vi "应变求平均.vi"(2 "调零采样数":u8=10, 3 "应变输入":dbl) -> (0 "调零-平均值":dbl, 1 "调零后应变值":dbl)   [LabVIEW 2019]
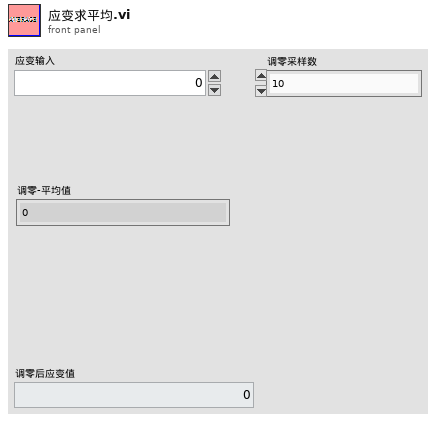
[diagram p1: front panel]
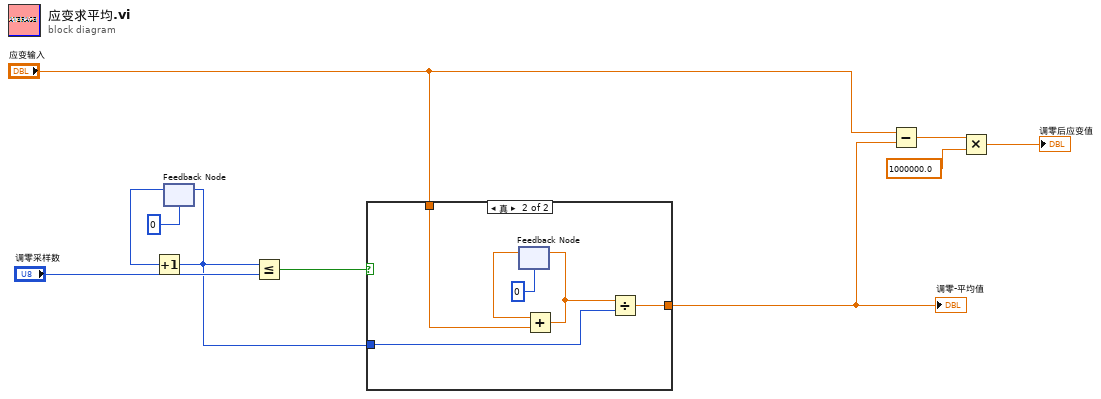
[diagram p0: block diagram]
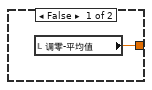
[diagram p2: hidden frame]
diagram:
  n1 = feedback #1(0) -> (w7:i32)
  n2 = Increment(x=w7) -> (x+1=w6:i32)
  n3 = feedback-in #1(w6) -> ()
  n4 = Less Or Equal?(x=w6, y="调零采样数") -> (x <= y?=w8:bool)
  n5 = case shown="真" w8 {
    tunnel: "应变输入" -> [_ w16]
    tunnel: w6 -> [_ w14]
    tunnel: [w11 w12] -> w4
    frame False {
      n6 = local read "调零-平均值"() -> (w11:dbl)
    }
    frame True {
      n7 = feedback #2(0) -> (w13:dbl)
      n8 = Add(x=w13, y=w16) -> (x+y=w15:dbl)
      n9 = feedback-in #2(w15) -> ()
      n10 = Divide(x=w15, y=w14) -> (x/y=w12:dbl)
    }
  }
  "调零-平均值" <- w4
  n11 = Subtract(x="应变输入", y=w4) -> (x-y=w3:dbl)
  n12 = Multiply(x=w3, y=1000000.0) -> (x*y=→"调零后应变值":dbl)
